vi "MotorFwdStop2sec.vi"   [LabVIEW 2012]
uses:
  <vilib>/NXT/Subs/MotorOutput.ctl
types:
  T1 = typedef "MotorOutput.ctl" = u8
  T2 = typedef "LVHSConnector.ctl" = refnum<class "BrickReference.lvclass">
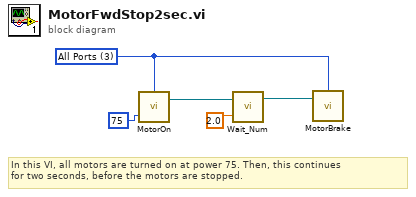
[diagram p0: block diagram]
diagram:
  w1 = T1 3 items=["Port A"=0, "Port B"=1, "Port C"=2, "Ports A & B"=4, "Ports A & C"=5, "Ports B & C"=6, "All Ports"=3] ("Output Port (All Ports)")
  # "In this VI, all motors are turned on at power 75. Then, this continues\nfor two seconds, before the motors are stopped."
  n1 = call <vilib>:"MotorOn.vi"("Power (75)"=75, "Output Port (All Ports)"=w1) -> ("NXT/EV3"=w5:T2)  [unwired: 2 in]
  n2 = call <vilib>:"Wait_Num.vi"("Time (1 sec)"=sgl 2.0, "NXT/EV3"=w5) -> ("NXT/EV3"=w4:T2)  [unwired: 2 in]
  n3 = call <vilib>:"MotorBrake.vi"("NXT/EV3"=w4, "Port (All Ports)"=w1) -> ()  [unwired: 2 in, 1 out]
